vi "Question Filiter.vi"(4 "Answer":T2, 6 "Question Index":T1, 11 "Classfy In":T3[](array[typedef])=[{"Item"="¤C¤H¨î¾ñÆV²y", "Count"=2, "Athletics"=["男子七人制橄欖球", "女子七人制橄欖球"]}, {"Item"="小輪車", "Count"=2, "Athletics"=["男子個人小輪車", "女子個人小輪車"]}, {"Item"="公路自由車", "Count"=4, "Athletics"=["女子計時賽公路自由車", "男子計時賽公路自由車", "男子公路賽公路自由車", "女子公路賽公路自由車"]}, {"Item"="手球", "Count"=2, "Athletics"=["男子手球", "女子手球"]}, {"Item"="¤ô¤WªÝÁ¢", "Count"=2, "Athletics"=["女子雙人水上芭蕾", "女子團體水上芭蕾"]}, {"Item"="水球", "Count"=2, "Athletics"=["男子水球", "女子水球"]}, {"Item"="¥Ð®|", "Count"=47, "Athletics"=["男子100公尺", "男子200公尺", "男子400公尺", "男子800公尺", "男子1500公尺", "男子5000公尺", "男子10,000公尺", "¨k¤l110¤½¤Ø¸óÄæ", "¨k¤l400¤½¤Ø¸óÄæ", "男子3000公尺障礙", "男子4×100公尺接力", "男子4×400公尺接力", "男子馬拉松", "男子20公里競走", "男子50公里競走", "男子跳高", "¨k¤l¼µ¬ñ¸õ°ª", "男子跳遠", "男子三級跳遠", "男子鉛球", "男子鐵餅", "男子鏈球", "男子標槍", "男子十項全能", "女子100公尺", "女子200公尺", "女子400公尺", "女子800公尺", "女子1500公尺", "女子5000公尺", "女子10,000公尺", "¤k¤l100¤½¤Ø¸óÄæ", "¤k¤l400¤½¤Ø¸óÄæ", "女子3000公尺障礙", "女子4×100公尺接力", "女子4×400公尺接力", "女子馬拉松", "女子20公里競走", "女子跳高", "¤k¤l¼µ¬ñ¸õ°ª", "女子跳遠", "女子三級跳遠", "女子鉛球", "女子鐵餅", "女子鏈球", "女子標槍", "女子七項全能"]}, {"Item"="¦E²î", "Count"=14, "Athletics"=["男子單人雙槳", "男子雙人單槳", "男子雙人雙槳", "男子四人單槳", "男子四人雙槳", "男子八人單槳", "男子輕量級雙人雙槳", "男子輕量級四人單槳", "女子單人雙槳", "女子雙人單槳", "女子雙人雙槳", "女子四人雙槳", "女子八人單槳", "女子輕量級雙人雙槳"]}, {"Item"="¦|²î", "Count"=10, "Athletics"=["¤k¤lRS¡GX«¬¡]­·®öªO¡^", "女子雷射輻射型（單人艇）", "女子470型（雙人艇）", "女子49人型FX（快艇）", "¨k¤lRS¡GX«¬¡]­·®öªO¡^", "男子雷射型（單人艇）", "男子芬蘭人型（單人艇）", "男子470型（雙人艇）", "男子49人型（快艇）", "混合Nacra17型（多體船）"]}, {"Item"="¦±´Ò²y", "Count"=2, "Athletics"=["男子曲棍球", "女子曲棍球"]}, {"Item"="¦Ð²y", "Count"=5, "Athletics"=["混合雙打羽球", "男子雙打羽球", "女子雙打羽球", "男子單打羽球", "女子單打羽球"]}, {"Item"="沙灘排球", "Count"=2, "Athletics"=["男子沙灘排球", "女子沙灘排球"]}, {"Item"="角力", "Count"=18, "Athletics"=["男子希羅式59公斤級", "男子希羅式66公斤級", "男子希羅式75公斤級", "男子希羅式85公斤級", "男子希羅式98公斤級", "男子希羅式130公斤級", "男子自由式57公斤級", "男子自由式65公斤級", "男子自由式74公斤級", "男子自由式86公斤級", "男子自由式97公斤級", "男子自由式125公斤級", "女子自由式48公斤級", "女子自由式53公斤級", "女子自由式58公斤級", "女子自由式63公斤級", "女子自由式69公斤級", "女子自由式75公斤級"]}, {"Item"="足球", "Count"=2, "Athletics"=["男子足球", "女子足球"]}, {"Item"="¬X¹D", "Count"=14, "Athletics"=["¨k¤l60¤½¤ç¯Å¬X¹D", "¨k¤l66¤½¤ç¯Å¬X¹D", "¨k¤l73¤½¤ç¯Å¬X¹D", "¨k¤l81¤½¤ç¯Å¬X¹D", "¨k¤l90¤½¤ç¯Å¬X¹D", "¨k¤l100¤½¤ç¯Å¬X¹D", "男子100公斤以上級柔道", "¤k¤l48¤½¤ç¯Å¬X¹D", "¤k¤l52¤½¤ç¯Å¬X¹D", "¤k¤l57¤½¤ç¯Å¬X¹D", "¤k¤l63¤½¤ç¯Å¬X¹D", "¤k¤l70¤½¤ç¯Å¬X¹D", "¤k¤l78¤½¤ç¯Å¬X¹D", "女子78公斤以上級柔道"]}, {"Item"="®g½b", "Count"=4, "Athletics"=["男子個人射箭", "女子個人射箭", "男子團體射箭", "女子團體射箭"]}, {"Item"="射擊", "Count"=15, "Athletics"=["男子10公尺空氣手槍", "男子10公尺空氣步槍", "男子25公尺快射手槍", "男子50公尺手槍", "¨k¤l50¤½¤Ø¨Bºjª×«º", "男子50公尺步槍三姿", "男子定向飛靶", "男子不定向飛靶", "男子雙不定向飛靶", "女子10公尺空氣手槍", "女子10公尺空氣步槍", "女子25公尺手槍", "女子50公尺步槍三姿", "女子定向飛靶", "女子不定向飛靶"]}, {"Item"="®±À»", "Count"=13, "Athletics"=["男子輕蠅量49公斤級", "¨k¤lÃÇ¶q52¤½¤ç¯Å", "¨k¤lÂú¶q56¤½¤ç¯Å", "男子輕量60公斤級", "男子輕沉量64公斤級", "¨k¤l¨I¶q69¤½¤ç¯Å", "男子中量75公斤級", "男子輕重量81公斤級", "男子重量91公斤級", "男子超重量91公斤以上級", "¤k¤lÃÇ¶q51¤½¤ç¯Å", "女子輕量60公斤級", "女子中量75公斤級"]}, {"Item"="桌球", "Count"=4, "Athletics"=["男子單打桌球", "女子單打桌球", "男子團體桌球", "女子團體桌球"]}, {"Item"="馬術", "Count"=6, "Athletics"=["團體盛裝舞步賽", "個人盛裝舞步賽", "個人三項賽", "團體三項賽", "團體場地障礙賽", "個人場地障礙賽"]}, {"Item"="高爾夫", "Count"=2, "Athletics"=["女子個人高爾夫", "男子個人高爾夫"]}, {"Item"="排球", "Count"=2, "Athletics"=["女子排球", "男子排球"]}, {"Item"="現代五項", "Count"=2, "Athletics"=["男子個人現代五項", "女子個人現代五項"]}, {"Item"="場地自由車", "Count"=10, "Athletics"=["男子團體爭先賽", "女子團體追逐賽", "男子團體追逐賽", "女子團體爭先賽", "男子爭先賽", "女子追逐賽", "男子追逐賽", "女子爭先賽", "男子全能", "女子全能"]}, {"Item"="´åªa", "Count"=34, "Athletics"=["男子捷泳：50公尺、100公尺、200公尺、400公尺、1500公尺", "女子捷泳：50公尺、100公尺、200公尺、400公尺、800公尺", "男子仰式：100公尺、200公尺", "女子仰式：100公尺、200公尺", "男子蛙式：100公尺、200公尺", "女子蛙式：100公尺、200公尺", "男子蝶式：100公尺、200公尺", "女子蝶式：100公尺、200公尺", "男子混合式：200公尺、400公尺", "女子混合式：200公尺、400公尺", "男子捷泳接力：4×100公尺、4×200公尺", "女子捷泳接力：4×100公尺、4×200公尺", "男子混合式接力：4×100公尺", "女子混合式接力：4×100公尺", "男子公開水域游泳：10公里", "女子公開水域游泳：10公里"]}, {"Item"="登山自由車", "Count"=2, "Athletics"=["男子越野賽", "女子越野賽"]}, {"Item"="¶`®±¹D", "Count"=8, "Athletics"=["¨k¤l58¤½¤ç¯Å¶`®±¹D", "¨k¤l68¤½¤ç¯Å¶`®±¹D", "¨k¤l80¤½¤ç¯Å¶`®±¹D", "¨k¤l80¤½¤ç¥H¤W¯Å¶`®±¹D", "¤k¤l49¤½¤ç¯Å¶`®±¹D", "¤k¤l57¤½¤ç¯Å ¶`®±¹D", "¤k¤l67¤½¤ç¯Å¶`®±¹D", "¤k¤l67¤½¤ç¥H¤W¯Å¶`®±¹D"]}, {"Item"="跳水", "Count"=8, "Athletics"=["女子3公尺跳板", "女子10公尺跳台", "女子雙人3公尺跳板", "女子雙人10公尺跳台", "男子3公尺跳板", "男子10公尺跳台", "男子雙人3公尺跳板", "男子雙人10公尺跳台"]}, {"Item"="網球", "Count"=5, "Athletics"=["女子單打網球", "女子雙打網球", "男子單打網球", "男子雙打網球", "混合雙打網球"]}, {"Item"="輕艇激流", "Count"=4, "Athletics"=["男子單人加拿大式艇", "男子雙人加拿大式艇", "男子單人愛斯基摩艇", "女子單人愛斯基摩艇"]}, {"Item"="輕艇競速", "Count"=12, "Athletics"=["男子200公尺單人加拿大式艇", "男子1000公尺單人加拿大式艇", "男子1000公尺雙人加拿大式艇", "男子200公尺單人愛斯基摩艇", "男子1000公尺單人愛斯基摩艇", "男子200公尺雙人愛斯基摩艇", "男子1000公尺雙人愛斯基摩艇", "男子1000公尺四人愛斯基摩艇", "女子500公尺單人愛斯基摩艇", "女子500公尺雙人愛斯基摩艇", "女子500公尺四人愛斯基摩艇", "女子200公尺單人愛斯基摩艇"]}, {"Item"="¼uÂ½§É", "Count"=2, "Athletics"=["男子個人彈翻床", "女子個人彈翻床"]}, {"Item"="À»¼C", "Count"=10, "Athletics"=["¤k¤l¶w¼C­Ó¤HÁÉ", "¨k¤l¶w¼C­Ó¤HÁÉ", "¨k¤l¶w¼C¹ÎÅéÁÉ", "¤k¤l¾U¼C­Ó¤HÁÉ", "¨k¤l¾U¼C­Ó¤HÁÉ", "¤k¤l¾U¼C¹ÎÅéÁÉ", "女子軍刀個人賽", "男子軍刀個人賽", "女子軍刀團體賽", "男子軍刀團體賽"]}, {"Item"="舉重", "Count"=15, "Athletics"=["男子56公斤級舉重", "男子62公斤級舉重", "男子69公斤級舉重", "男子77公斤級舉重", "男子85公斤級舉重", "男子94公斤級舉重", "男子105公斤級舉重", "男子105公斤以上級舉重", "女子48公斤級舉重", "女子53公斤級舉重", "女子58公斤級舉重", "女子63公斤級舉重", "女子69公斤級舉重", "女子75公斤級舉重", "女子75公斤以上級舉重"]}, {"Item"="韻律體操", "Count"=2, "Athletics"=["女子個人全能韻律體操", "女子團體全能韻律體操"]}, {"Item"="競技體操", "Count"=14, "Athletics"=["男子個人全能競技體操", "男子團體競技體操", "男子跳馬", "男子自由體操", "男子鞍馬", "男子吊環", "男子雙槓", "男子單槓", "女子個人全能競技體操", "女子團體競技體操", "女子跳馬", "女子平衡木", "女子高低槓", "女子自由體操"]}, {"Item"="Äx²y", "Count"=2, "Athletics"=["男子籃球", "女子籃球"]}, {"Item"="鐵人三項", "Count"=2, "Athletics"=["男子個人鐵人三項", "女子個人鐵人三項"]}]) -> (3 "Classfy Out":T3[](array[typedef])=[{"Item"="¤C¤H¨î¾ñÆV²y", "Count"=2, "Athletics"=["男子七人制橄欖球", "女子七人制橄欖球"]}, {"Item"="手球", "Count"=2, "Athletics"=["男子手球", "女子手球"]}, {"Item"="水球", "Count"=2, "Athletics"=["男子水球", "女子水球"]}, {"Item"="¦±´Ò²y", "Count"=2, "Athletics"=["男子曲棍球", "女子曲棍球"]}, {"Item"="¦Ð²y", "Count"=5, "Athletics"=["混合雙打羽球", "男子雙打羽球", "女子雙打羽球", "男子單打羽球", "女子單打羽球"]}, {"Item"="沙灘排球", "Count"=2, "Athletics"=["男子沙灘排球", "女子沙灘排球"]}, {"Item"="足球", "Count"=2, "Athletics"=["男子足球", "女子足球"]}, {"Item"="桌球", "Count"=4, "Athletics"=["男子單打桌球", "女子單打桌球", "男子團體桌球", "女子團體桌球"]}, {"Item"="排球", "Count"=2, "Athletics"=["女子排球", "男子排球"]}, {"Item"="網球", "Count"=5, "Athletics"=["女子單打網球", "女子雙打網球", "男子單打網球", "男子雙打網球", "混合雙打網球"]}, {"Item"="Äx²y", "Count"=2, "Athletics"=["男子籃球", "女子籃球"]}])   [LabVIEW 2015]
uses:
  Data Def/Classify.ctl
  Data Def/Answer.ctl
  Data Def/Question Index.ctl
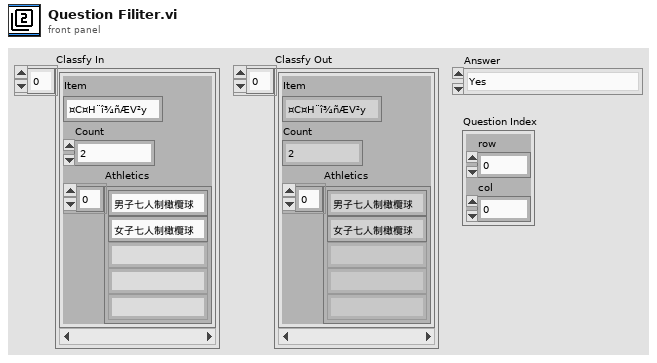
[diagram p1: front panel]
types:
  T1 = typedef "Question Index.ctl" = cluster{"row":i32, "col":i32}
  T2 = typedef "Answer.ctl" = enum16{"Yes", "No", "I don't Know"}
  T3 = typedef "Classify.ctl" = cluster{"Item":string, "Count":i32, "Athletics":string[]}
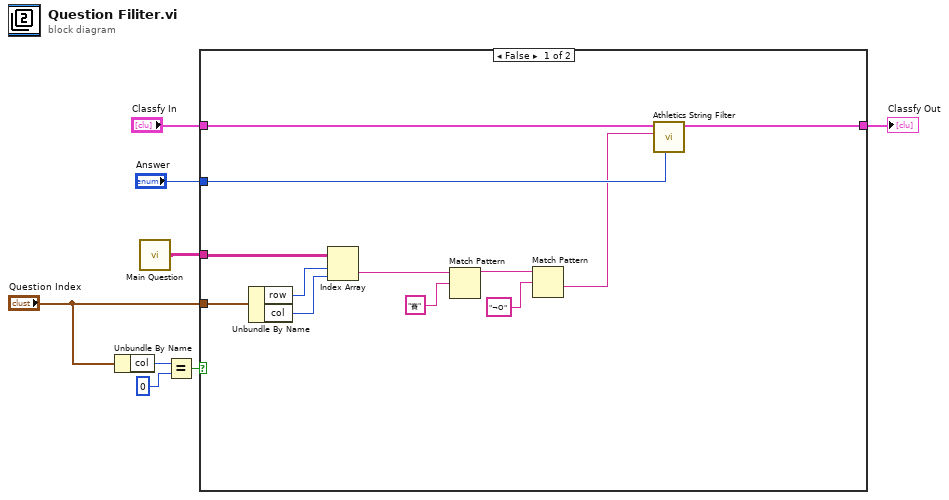
[diagram p0: block diagram]
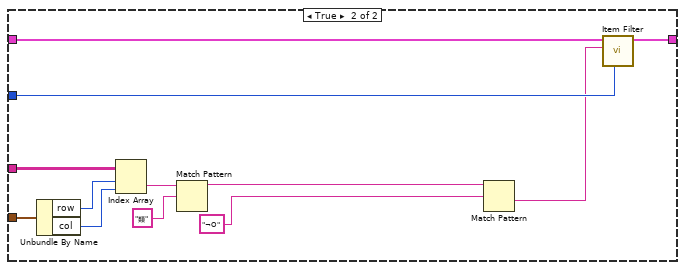
[diagram p2: hidden frame]
diagram:
  n1 = Unbundle By Name("Question Index") -> ("col"=w8:i32)
  n2 = call "Main Question.vi"() -> ("Question"=w1:string[][])
  n3 = Equal?(x=w8, y=0) -> (x = y?=w6:bool)
  n4 = case shown="False" w6 {
    tunnel: "Question Index" -> [w17 w32]
    tunnel: "Classfy In" -> [w16 w29]
    tunnel: "Answer" -> [w10 w28]
    tunnel: [w15 w27] -> w2
    tunnel: w1 -> [w18 w21]
    frame False {
      n5 = Unbundle By Name(w17) -> ("row"=w20:i32, "col"=w19:i32)
      n6 = Index Array(array=w18, index (row)=w20, index (col)=w19) -> (element=w13:string)
      n7 = Match Pattern(string=w13, regular expression="賽") -> (before substring=w12:string)  [unwired: 1 in, 3 out]
      n8 = Match Pattern(string=w12, regular expression="¬O") -> (after substring=w9:string)  [unwired: 1 in, 3 out]
      n9 = call "Athletics String Filter.vi"("Answer"=w10, "Match String"=w9, "Classfy In"=w16) -> ("Classfy Out"=w15:T3[])  [unwired: 8 in]
    }
    frame True {
      n10 = Unbundle By Name(w32) -> ("row"=w31:i32, "col"=w30:i32)
      n11 = Index Array(array=w21, index (row)=w31, index (col)=w30) -> (element=w26:string)
      n12 = Match Pattern(string=w26, regular expression="類") -> (before substring=w24:string)  [unwired: 1 in, 3 out]
      n13 = Match Pattern(string=w24, regular expression="¬O") -> (after substring=w22:string)  [unwired: 1 in, 3 out]
      n14 = call "Item Filter.vi"("Answer"=w28, "Item"=w22, "Classfy In"=w29) -> ("Classfy Out"=w27:T3[])  [unwired: 8 in]
    }
  }
  "Classfy Out" <- w2
